vi "Pre Launch Init.vi"(11 "BuildWorker in":refnum<class "BuildWorker.lvclass">) -> (0 "error out":errorcluster, 3 "BuildWorker out":refnum<class "BuildWorker.lvclass">)   [LabVIEW 2017, in "BuildWorker.lvlib" / "BuildWorker.lvclass"]
doc: "(<B>Filename</B>: Actor Framework.lvlib:Actor.lvclass:Pre Launch Init.vi)\n\nDefines behavior that occurs after the Launch Nested Actor method is invoked but before the actor's Actor Core method begins running.\n\nBy default, this method does nothing. A descendant class may override it to define behavior."
uses:
  BuildWorker.lvclass
  Events.ctl
  BuildWorker.lvclass/BuildWorker.ctl
  Framework/Actor wUI/Actor wUI.lvclass
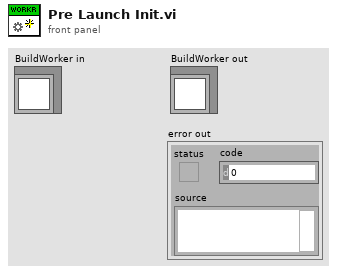
[diagram p1: front panel]
types:
  T1 = typedef "BuildWorker.lvlib/BuildWorker.lvclass/Events.ctl" = cluster{"Stop":refnum<user-event>}
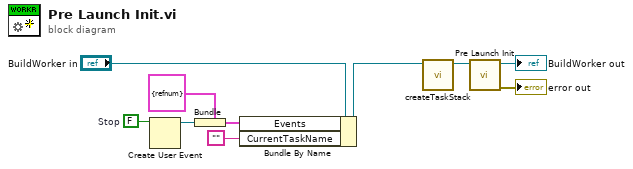
[diagram p0: block diagram]
diagram:
  w7 = FALSE  # Stop
  n1 = Create User Event(user event datatype=w7) -> (user event=w6:refnum<user-event>)  [unwired: 1 in, 1 out]
  n2 = Bundle(cluster=T1 {"Stop"=refnum} ("Events"), "Stop"=w6) -> (w4:T1)
  n3 = Bundle By Name(cluster="BuildWorker in", "Events"=w4, "CurrentTaskName"="") -> (w1:refnum<class "BuildWorker.lvclass">)
  n4 = call "createTaskStack.vi"("BuildWorker in"=w1) -> ("BuildWorker out"=w3:refnum<class "BuildWorker.lvclass">)  [unwired: 9 in, 1 out]
  n5 = call-parent "Pre Launch Init.vi"("Actor in"=w3) -> ("error out"=→"error out":errorcluster, "Actor out"=→"BuildWorker out":refnum<class "BuildWorker.lvclass">)  [unwired: 9 in]
